vi "re-init on shoot.vi"(1 "Value":T1=enum."Forward") -> (0 "Value":T1=enum."Forward")   [LabVIEW 2013]
uses:
  <vilib>/Rock Robotics/WPI/Solenoid/WPI_SolenoidValue.ctl
  typedefs/fg_typedef.ctl
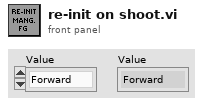
[diagram p1: front panel]
types:
  T1 = typedef "WPI_SolenoidValue.ctl" = enum16{"Off", "On", "Forward", "Reverse"}
  T2 = typedef "fg_typedef.ctl" = enum16{"Get", "Set"}
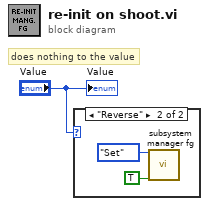
[diagram p0: block diagram]
diagram:
  # "does nothing to the value"
  n1 = case shown="\"Reverse\"" "Value" {
    frame "Off", Default {
    }
    frame "Reverse" {
      n2 = call "subsystem manager fg.vi"("Menu"=fg_typedef."Set", "Re-Initalize"=TRUE) -> ()  [unwired: 13 in, 5 out]
    }
  }
  "Value" <- "Value"
